vi "niDTS Calibration Cal IsNeeded RF Test Full Example.vi"() -> ()   [LabVIEW 2014]
uses:
  Cal IsNeeded RF Test/Includes/niDTS Calibration Cal IsNeeded RF Test INC Parameters.ctl
  Cal IsNeeded RF Test/Includes/niDTS Calibration Cal IsNeeded RF Test INC Results.ctl
  TestStand/Station/Objects/SystemDutHandle/Includes/niDTS SystemDutHandle INC SystemDutHandles.ctl
  TestStand/Station/Objects/SystemDutHandle/niDTS SystemDutHandle.lvclass
  Framework/Dut/Includes/niDTS Dut INC Handle.ctl
  Framework/Dut/Objects/BASE_class/niDTS Dut.lvclass
  TestStand/Station/Objects/SystemTechnologyCatalog/niDTS SystemTechnologyCatalog.lvclass
  TestStand/Station/Objects/SystemDut/niDTS SystemDut.lvclass
  Framework/niDTS Framework.lvlib
  TestStand/niDTS TestStand.lvlib
  Plugins/niWTM Loopback/niWTM Loopback.lvlib
  Framework/Logger/Listener/Viewer/niDTS Logger Listener Viewer.lvclass
  niDTS Utilities.lvlib
panel:
  in  "Results":enum32{"Calibration"}(tab)
  out "Results":T1
  in  "Keep Log Open":bool
  in  "ResultsIndex":u8=1
  in  "System Configuration XML Path":path=path "C:/Users/Public/Documents/National Instruments/WTM 1.0/System Configurations"
  in  "Socket Index":i32
  out "error out":errorcluster
  in  "DUT Config":enum32{"Loopback"}(tab)
  in  "Socket Parameters":T2={"Calibration"={"VISA Resource"="TCPIP0::InstrumentAddress::inst0::INSTR", "PortNames "=["Port0"]}}
  in  "Test Config":enum32{"Calibration"}(tab)
  in  "Parameters":T3={"Temperature Change"=2.0, "Time Range"=24}
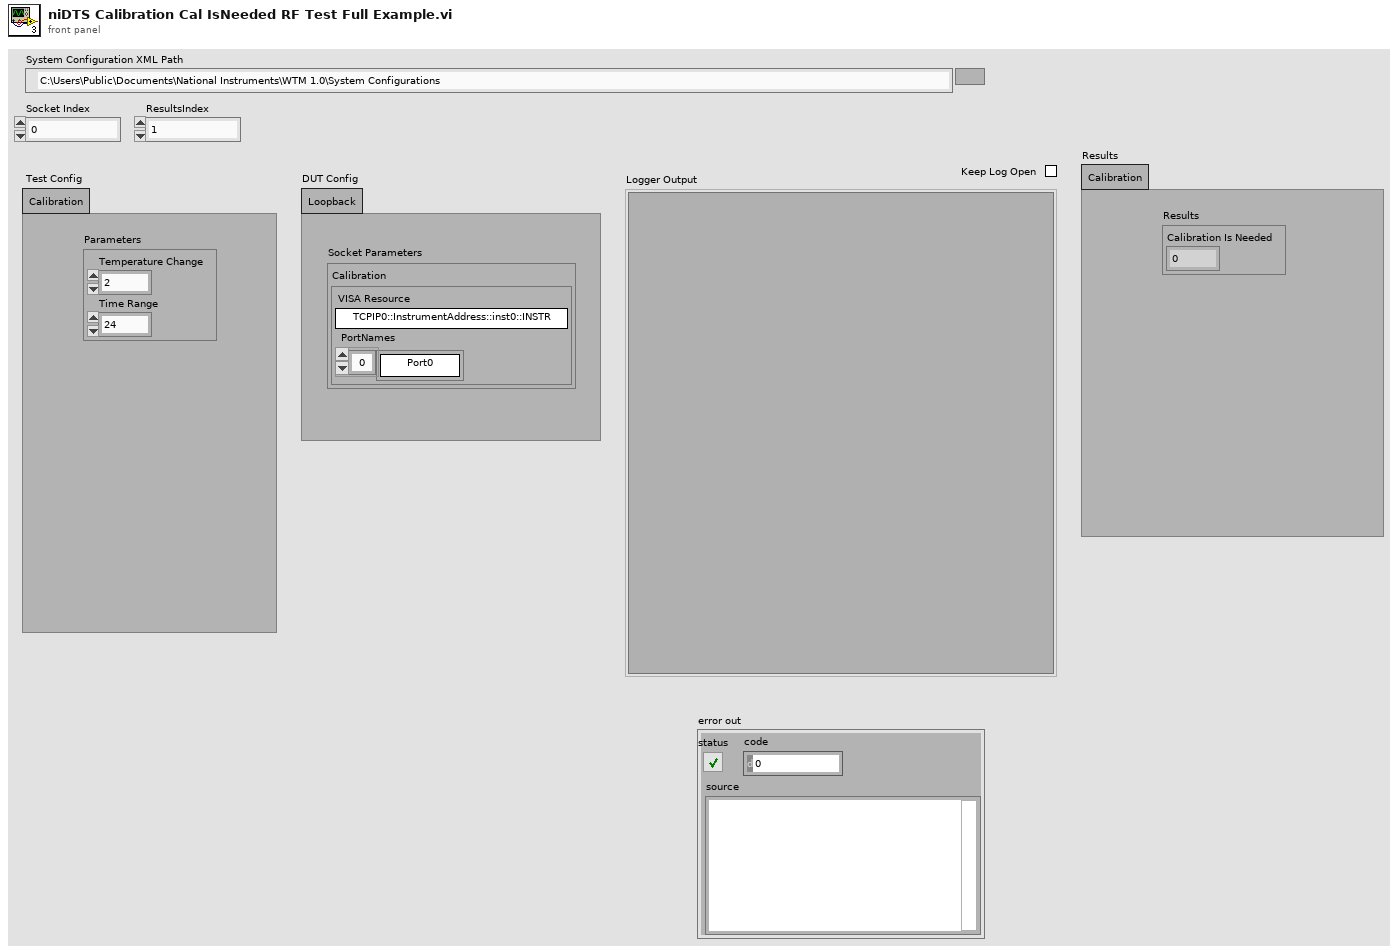
[diagram p1: front panel]
types:
  T1 = typedef "niDTS Utilities.lvlib/niDTS Calibration Cal IsNeeded RF Test INC Results.ctl" = cluster{"Calibration Is Needed":u8}
  T2 = cluster{"Calibration":cluster{"VISA Resource":string, "PortNames ":string[]}}
  T3 = typedef "niDTS Utilities.lvlib/niDTS Calibration Cal IsNeeded RF Test INC Parameters.ctl" = cluster{"Temperature Change":dbl, "Time Range":i32}
  T4 = cluster{"WLAN":cluster{"VISA Resource":string, "PortNames ":string[]}, "Bluetooth":cluster{"VISA Resource":string, "PortNames ":string[]}, "GNSS":cluster{"VISA Resource":string, "PortNames ":string[]}}
  T5 = cluster{"WLAN":cluster{"idle interval":dbl, "Payload Length Limit":i32, "Channel Secondary Factor":enum16{"-1", "1", "0"}}}
  T6 = typedef "niDTS Framework.lvlib/niDTS Dut INC Handle.ctl" = refnum<data-value>
  T7 = typedef "niDTS TestStand.lvlib/niDTS SystemDutHandle.lvclass/niDTS SystemDutHandle INC SystemDutHandles.ctl" = refnum<class "niDTS SystemDutHandle.lvclass">[]
  T8 = typedef "niDTS Framework.lvlib/niDTS Logger INC Handle.ctl" = refnum<data-value>
  T9 = cluster{"VISA Resource":string, "PortNames ":string[]}
  T10 = typedef "niDTS Utilities.lvlib/niDTS Calibration Cal IsNeeded RF Test INC Handle.ctl" = refnum<data-value>
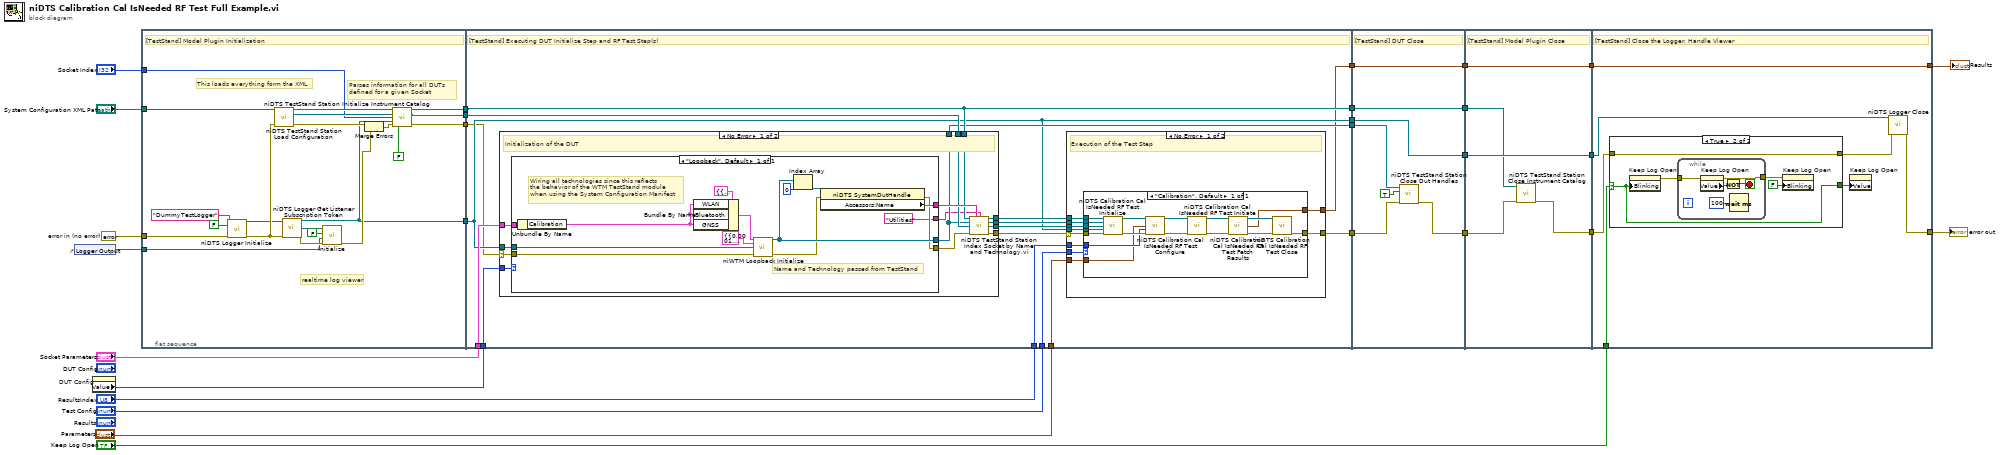
[diagram p0: block diagram]
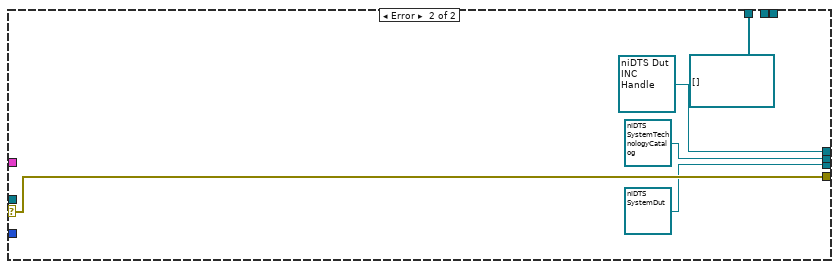
[diagram p2: hidden frame]
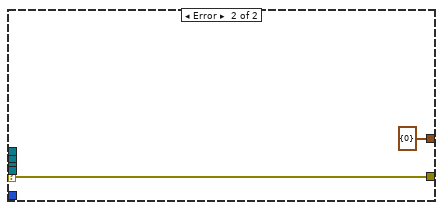
[diagram p3: hidden frame]
diagram:
  w22 = errorcluster {"status"=FALSE, "code"=0, "source"=""}  # error in (no error)
  n1 = control-ref of="Logger Output"() -> (w21:refnum<vi>)
  n2 = property on="DUT Config" class="TabCtl (strict)"() -> ("Value"=w8:enum32{"Loopback"})  [unwired: 2 in, 2 out]
  n3 = flat-sequence {
    tunnel: [w36] -> w28
    tunnel: [w35] -> w27
    tunnel: [w34] -> w26
    tunnel: [w33] -> w25
    tunnel: "Socket Index" -> [w32]
    tunnel: "System Configuration XML Path" -> [w31]
    tunnel: w22 -> [w30]
    tunnel: w21 -> [w29]
    tunnel: w28 -> [w61]
    tunnel: w27 -> [w62]
    tunnel: w26 -> [w51]
    tunnel: w25 -> [w56]
    tunnel: "Socket Parameters" -> [w60]
    tunnel: w8 -> [w59]
    tunnel: [w61] -> w20
    tunnel: [w58] -> w18
    tunnel: [w57] -> w16
    tunnel: [w56] -> w15
    tunnel: "ResultsIndex" -> [w53]
    tunnel: "Test Config" -> [w55]
    tunnel: "Parameters" -> [w54]
    tunnel: [w50] -> w4
    tunnel: w20 -> [w134]
    tunnel: [w134] -> w19
    tunnel: w18 -> [w130]
    tunnel: [w129] -> w17
    tunnel: w16 -> [w131]
    tunnel: w15 -> [w133]
    tunnel: [w133] -> w14
    tunnel: [w128] -> w5
    tunnel: w4 -> [w128]
    tunnel: w19 -> [w137]
    tunnel: w17 -> [w136]
    tunnel: w14 -> [w139]
    tunnel: [w139] -> w13
    tunnel: [w138] -> w12
    tunnel: [w135] -> w6
    tunnel: w5 -> [w135]
    tunnel: [w143] -> w11
    tunnel: w13 -> [w146]
    tunnel: w12 -> [w144]
    tunnel: "Keep Log Open" -> [w142]
    tunnel: w6 -> [w141]
    tunnel: [w141] -> w2
    frame #0 {
      # "realtime log viewer"
      # "Parses information for all DUTs defined for a given Socket"
      # "This loads everything form the XML"
      # "[TestStand] Model Plugin Initialization"
      n4 = call "niDTS Logger Initialize.vi"("Session Name ()"="DummyTestLogger", "Log to File"=FALSE, "error in (no error)"=w30) -> ("Logger Handle out"=w45:T8, "error out"=w46:errorcluster)  [unwired: 11 in]
      n5 = call "niDTS TestStand Station Load Configuration.vi"("System Configuration XML Path"=w31, "error in (no error)"=w46) -> ("All System Hardware"=w41:refnum<class "niDTS SystemHardware.lvclass">, "All DUT Definitions"=w39:refnum<class "niDTS SystemDut.lvclass">[], "error out"=w48:errorcluster)  [unwired: 11 in]
      n6 = call "niDTS Logger Get Listener Subscription Token.vi"("Logger Handle in"=w45, "error in (no error)"=w46) -> ("Logger Handle out"=w33:T8, "Listener Subscription Token"=w42:refnum<class "niDTS Logger Listener Subscription Token.lvclass">, "error out"=w43:errorcluster)  [unwired: 11 in]
      n7 = call "Initialize.vi"("error in (no error)"=w43, "SubPanel Reference"=w29, "Open Viewer?"=FALSE, "Listener Subscription Token"=w42) -> ("error out"=w49:errorcluster)  [unwired: 6 in, 1 out]
      n8 = Merge Errors(w48, w49) -> (w47:errorcluster)
      n9 = call "niDTS TestStand Station Initialize Instrument Catalog.vi"("All System Hardware"=w41, "All DUT Definitions"=w39, "Socket Index"=w32, "Logger Handle"=w33, "error in (no error)"=w47, "Simulation Mode (F)"=FALSE) -> ("Socket Instrument Catalog"=w36:refnum<class "niDTS SystemInstrCatalog.lvclass">, "Socket DUT Definitions"=w35:refnum<class "niDTS SystemDut.lvclass">[], "error out"=w34:errorcluster)  [unwired: 7 in]
    }
    frame #1 {
      # "[TestStand] Executing DUT Initialize Step and RF Test Step(s)"
      n10 = case shown="No Error" w51 {
        selector: w51 -> [w67 w98]
        tunnel: [w78 refnum<class "niDTS SystemDut.lvclass"> refnum ("Specific Socket/Tech DUT Definition")] -> w65
        tunnel: [w77 refnum<class "niDTS SystemTechnologyCatalog.lvclass"> refnum ("SystemTechnologyCatalog")] -> w64
        tunnel: [w76 T6 refnum ("Dut Handle")] -> w63
        tunnel: w62 -> [w75 _]
        tunnel: w61 -> [w74 _]
        tunnel: w60 -> [w73 _]
        tunnel: w59 -> [w72 _]
        tunnel: [w71 T7 [] ("Dut Technology Handles")] -> w57
        tunnel: w56 -> [w70 _]
        tunnel: [w69 w98] -> w52
        frame No Error {
          # "Initialization of the DUT"
          n11 = case shown="\"Loopback\", Default" w72 {
            tunnel: [w87] -> w68
            tunnel: w70 -> [w86]
            tunnel: [w90] -> w71
            tunnel: [w89] -> w79
            tunnel: w73 -> [w81]
            tunnel: w67 -> [w85]
            tunnel: ["Utilities"] -> w66
            frame "Loopback", Default {
              # "Wiring all technologies since this reflects \nthe behavior of the WTM TestStand module \nwhen using the System Configuration Manifest"
              # "Name and Technology passed from TestStand"
              n12 = Unbundle By Name(w81) -> ("Calibration"=w80:T9)
              n13 = Bundle By Name(cluster=T4 {"WLAN"={"VISA Resource"="TCPIP0::InstrumentAddress::inst0::INSTR", "PortNames "=["Port0"]}, "Bluetooth"={"VISA Resource"="TCPIP0::InstrumentAddress::inst0::INSTR", "PortNames "=["Port0"]}, "GNSS"={"VISA Resource"="TCPIP0::InstrumentAddress::inst0::INSTR", "PortNames "=["Port0"]}} ("Socket Parameters"), "WLAN"=w80, "Bluetooth"=w80, "GNSS"=w80) -> (w82:T4)
              n14 = call "niWTM Loopback Initialize.vi"("Socket Parameters"=w82, "General Parameters"=T5 {"WLAN"={"idle interval"=0.0001, "Payload Length Limit"=12000, "Channel Secondary Factor"=enum."0"}} ("General Parameters niWTM Loopback"), "Logger"=w86, "error in (no error)"=w85) -> ("Dut Technology Handles"=w90:T7, "error out"=w88:errorcluster)  [unwired: 10 in]
              n15 = Index Array(array=w90, index=0) -> (element=w91:refnum<class "niDTS SystemDutHandle.lvclass">)
              n16 = property class="niDTS SystemDutHandle"(reference=w91, error in=w88) -> (error out=w87:errorcluster, "Accessors:Name"=w89:string)  [unwired: 1 out]
            }
          }
          n17 = call "niDTS TestStand Station Index Socket by Name and Technology,vi.vi"("niDTS SystemInstrCatalog in"=w74, "Name"=w79, "Technology"=w66, "System Dut Handles"=w71, "Socket DUT Definitions"=w75, "error in (no error)"=w68) -> ("Dut Handle"=w76:T6, "SystemTechnologyCatalog"=w77:refnum<class "niDTS SystemTechnologyCatalog.lvclass">, "Specific Socket/Tech DUT Definition"=w78:refnum<class "niDTS SystemDut.lvclass">, "error out"=w69:errorcluster)  [unwired: 6 in]
        }
        frame Error {
        }
      }
      n18 = case shown="No Error" w52 {
        selector: w52 -> [w100 w127]
        tunnel: w65 -> [w108 _]
        tunnel: w64 -> [w107 _]
        tunnel: w63 -> [w106 _]
        tunnel: [w105 w127] -> w58
        tunnel: w56 -> [w104 _]
        tunnel: w55 -> [w103 _]
        tunnel: w54 -> [w102 _]
        tunnel: w53 -> [w101 _]
        tunnel: [w99 T1 {"Calibration Is Needed"=0} ("Results")] -> w50
        frame No Error {
          # "Execution of the Test Step"
          n19 = case shown="\"Calibration\", Default" w103 {
            tunnel: [w111] -> w105
            tunnel: w100 -> [w125]
            tunnel: w104 -> [w124]
            tunnel: w106 -> [w121]
            tunnel: w107 -> [w122]
            tunnel: w108 -> [w123]
            tunnel: w101 -> [w118]
            tunnel: [w109] -> w99
            tunnel: w102 -> [w110]
            frame "Calibration", Default {
              n20 = call "niDTS Calibration Cal IsNeeded RF Test Initialize.vi"("Dut Reference"=w121, "SystemTechnologyCatalog"=w122, "SystemDut"=w123, "Logger Reference"=w124, "error in (no error)"=w125) -> ("Template Tx Test Handle"=w120:T10, "error out"=w119:errorcluster)  [unwired: 8 in, 1 out]
              n21 = call "niDTS Calibration Cal IsNeeded RF Test Configure.vi"("Template Tx Test Handle in"=w120, "Parameters"=w110, "ResultsIndex"=w118, "error in (no error)"=w119) -> ("Template Tx Test Handle out"=w117:T10, "error out"=w116:errorcluster)  [unwired: 10 in]
              n22 = call "niDTS Calibration Cal IsNeeded RF Test Initiate.vi"("Template Tx Test Handle in"=w117, "error in (no error)"=w116) -> ("Template Tx Test Handle out"=w114:T10, "error out"=w115:errorcluster)  [unwired: 12 in]
              n23 = call "niDTS Calibration Cal IsNeeded RF Test Fetch Results.vi"("Template Tx Test Handle in"=w114, "error in (no error)"=w115) -> ("Template Tx Test Handle out"=w113:T10, "Results"=w109:T1, "error out"=w112:errorcluster)  [unwired: 11 in]
              n24 = call "niDTS Calibration Cal IsNeeded RF Test Close.vi"("Template Tx Test Handle"=w113, "error in (no error)"=w112) -> ("error out"=w111:errorcluster)  [unwired: 13 in]
            }
          }
        }
        frame Error {
        }
      }
    }
    frame #2 {
      # "[TestStand] DUT Close"
      n25 = call "niDTS TestStand Station Close Dut Handles.vi"("Socket Dut Handles In"=w131, "Close All"=TRUE, "error in (no error)"=w130) -> ("error out"=w129:errorcluster)  [unwired: 11 in, 1 out]
    }
    frame #3 {
      # "[TestStand] Model Plugin Close"
      n26 = call "niDTS TestStand Station Close Instrument Catalog.vi"("Socket Instrument Catalog"=w137, "error in (no error)"=w136) -> ("error out"=w138:errorcluster)  [unwired: 13 in]
    }
    frame #4 {
      # "[TestStand] Close the Logger. Handle Viewer"
      n27 = case shown="True" w142 {
        selector: w142 -> [w147 w149]
        tunnel: w144 -> [w148 w153]
        tunnel: [w148 w153] -> w145
        tunnel: [w147 w149] -> w140
        frame False {
        }
        frame True {
          n28 = property on="Keep Log Open" class="Bool (strict)"("Blinking"=w149) -> (error out=w150:errorcluster)  [unwired: 2 in, 1 out]
          n29 = while {
            tunnel: [w157] -> w151
            tunnel: w150 -> [w156]
            stop <- w155 stop-if-true
            n30 = property on="Keep Log Open" class="Bool (strict)"(error in=w156) -> (error out=w157:errorcluster, "Value"=w154:bool)  [unwired: 1 in, 1 out]
            n31 = Not(x=w154) -> (.not. x?=w155:bool)
            n32 = Wait (ms)(milliseconds to wait=u32 100) -> ()  [unwired: 1 out]
          }
          n33 = property on="Keep Log Open" class="Bool (strict)"(error in=w151, "Blinking"=FALSE) -> ()  [unwired: 1 in, 2 out]
        }
      }
      n34 = property on="Keep Log Open" class="Bool (strict)"("Value"=w140) -> ()  [unwired: 2 in, 2 out]
      n35 = call "niDTS Logger Close.vi"("Logger Handle in"=w146, "error in (no error)"=w145) -> ("error out"=w143:errorcluster)  [unwired: 13 in]
    }
  }
  "error out" <- w11
  "Results" <- w2
